vi "TriangleSubVI.vi"(6 "Error In":errorcluster, 8 "Frequency":dbl, 9 "DC Offset":dbl, 10 "Duty Cycle":dbl, 11 "Amplitude":dbl) -> (0 "Error Out":errorcluster, 3 "Array":dbl[](array[numeric]))   [LabVIEW 2017]
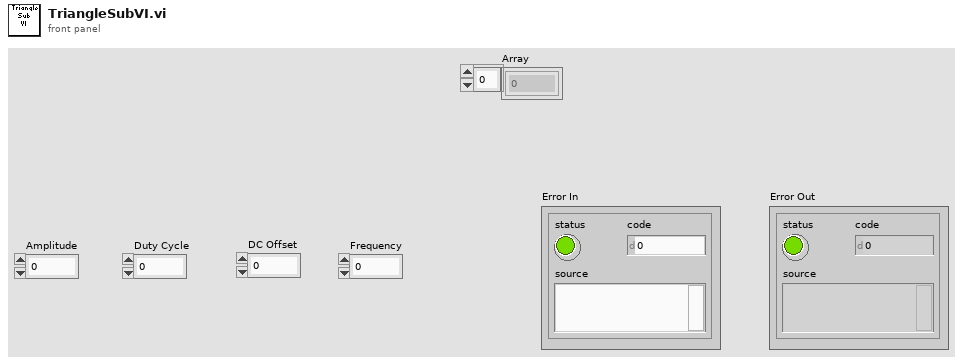
[diagram p1: front panel]
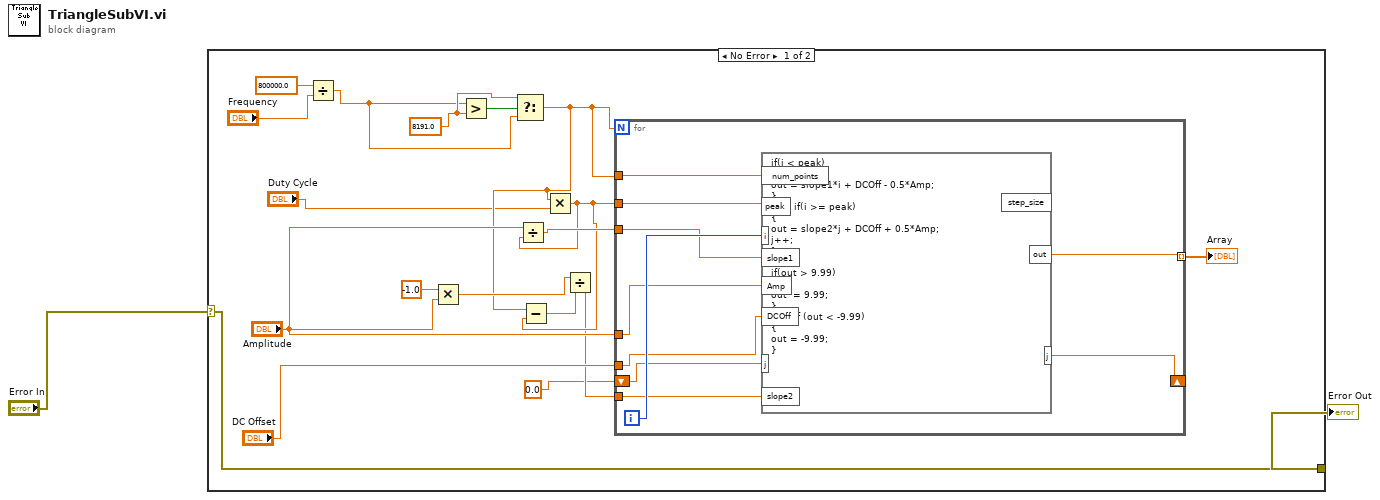
[diagram p0: block diagram]
diagram:
  n1 = case shown="No Error" "Error In" {
    selector: "Error In" -> [w20 w31]
    tunnel: [w20 w31] -> w1
    frame No Error {
      w16 = 8191.0 ("y")
      n2 = Divide(x=800000.0, y="Frequency") -> (x/y=w15:dbl)
      n3 = Multiply(x=-1.0, y="Amplitude") -> (x*y=w10:dbl)
      n4 = Greater?(x=w15, y=w16) -> (0:w19:bool)
      n5 = Select(t=w16, s=w19, f=w15) -> (s? t:f=w9:dbl)
      n6 = Multiply(x=w9, y="Duty Cycle") -> (x*y=w8:dbl)
      n7 = Divide(x="Amplitude", y=w8) -> (x/y=w13:dbl)
      n8 = Subtract(x=w9, y=w8) -> (x-y=w7:dbl)
      n9 = Divide(x=w10, y=w7) -> (x/y=w6:dbl)
      n10 = for {
        N: w9 -> [_]
        tunnel: w8 -> [w30]
        tunnel: "Amplitude" -> [w28]
        tunnel: "DC Offset" -> [w27]
        tunnel: w9 -> [w26]
        tunnel: w13 -> [w25]
        tunnel: w6 -> [w24]
        tunnel: [w23] -> w5 mode=indexing
        shift-right: [w22] -> _
        shift-left: 0.0 -> [w21]
        i -> [w29]
        n11 = formula code="if(i < peak)\n{\nout = slope1*i + DCOff - 0.5*Amp;\n}\nelse if(i >= peak)\n{\nout = slope2*j + DCOff + 0.5*Amp;\nj++;\n}\n\nif(out > 9.99)\n{\nout  = 9.99;\n}\nelse if (out < -9.99)\n{\nout = -9.99;\n}"("peak"=w30, "i"=w29, "Amp"=w28, "DCOff"=w27, "num_points"=w26, "slope1"=w25, "slope2"=w24, "j"=w21) -> ("out"=w23:dbl, "j"=w22:dbl)  [unwired: 1 out]
      }
      "Array" <- w5
    }
    frame Error {
    }
  }
  "Error Out" <- w1
